vi "WPI_IMU_ADIS16448_Loop.vi"(8 "error in":errorcluster, 11 "ADI IMU Interrupt DevRef":T1={"ADI IMU DevRef"={"DevStatus"={"status"=FALSE, "code"=0, "source"=""}, "Handle"=0, "SPI Bus"=enum."SPI On-Board, CS0", "Device Found"=FALSE, "Device Ready"=FALSE, "Yaw Axis"=enum."Z", "AHRS Algorithm"=enum."Complementary", "Serial"=0, "Lot ID 2"=0, "Lot ID 1"=0, "Product ID"=0}, "InterruptRef"={"DevStatus"={"status"=FALSE, "code"=0, "source"=""}, "InterruptIndex"=enum."0"}}) -> (0 "error out":errorcluster, 1 "Device Found":bool)   [LabVIEW 2015, in "Apple Pi Gyro Library.lvlib" / "FRC_ADIS16448_IMU.lvlib"]
doc: "Periodically reads the ADI MXP IMU valuse and makes data available for use elsewhere in your robot project. Place this block within PeriodicTasks.vi outside any loops."
uses:
  FRC_ADIS16448_IMU.lvlib
  WPI_IMU_ADIS16448_InterruptDevRef.ctl
  WPI_IMU_ADIS16448_IMUDevRef.ctl
  <vilib>/Rock Robotics/SystemInterfaces/spilib/spi_bus.ctl
  <vilib>/Rock Robotics/WPI/Interrupt/WPI_InterruptRef.ctl
  <vilib>/Rock Robotics/SystemInterfaces/Interrupt/FPGA_InterruptIndex.ctl
  <vilib>/Rock Robotics/WPI/SPI/WPI_SPIDevRef.ctl
  WPI_IMU_ADIS16448_Registers.ctl
  <vilib>/Platform/TimedLoop/XDataNode/timing_clust.ctl
  <vilib>/Platform/TimedLoop/XDataNode/nitl_modes.ctl
  <vilib>/Platform/TimedLoop/XDataNode/wakeup.ctl
  <vilib>/Rock Robotics/SystemInterfaces/Utilities/FPGA_UtilitiesRead LocalTime.vi
  <vilib>/Rock Robotics/SystemInterfaces/Interrupt/FPGA_WaitOnInterrupt.vi
  <vilib>/Rock Robotics/WPI/Utilities/WPI_UtilitiesTimebaseConstants.vi
  <vilib>/Rock Robotics/SystemInterfaces/Interrupt/FPGA_InterruptReadTimestamp.vi
  <vilib>/platform/TimedLoop/XDataNode/XDataNode.xnode
  <vilib>/Platform/TimedLoop/XDataNode/XDNodeRunTimeDep.lvlib
  <vilib>/ptbypt/NI_PtbyPt.lvlib
panel:
  out "SPS":dbl
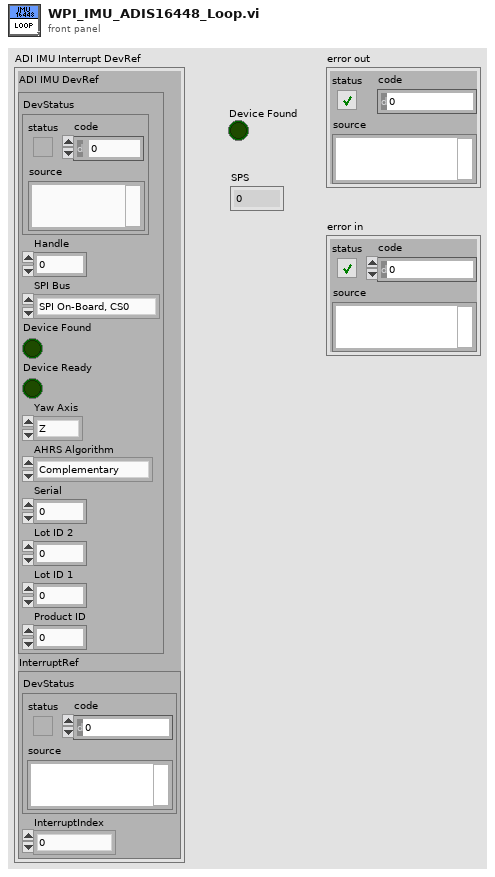
[diagram p1: front panel]
types:
  T1 = typedef "Apple Pi Gyro Library.lvlib/FRC_ADIS16448_IMU.lvlib/WPI_IMU_ADIS16448_InterruptDevRef.ctl" = cluster{"ADI IMU DevRef":T2, "InterruptRef":T4}
  T2 = typedef "Apple Pi Gyro Library.lvlib/FRC_ADIS16448_IMU.lvlib/WPI_IMU_ADIS16448_IMUDevRef.ctl" = cluster{"DevStatus":errorcluster, "Handle":i32, "SPI Bus":T3, "Device Found":bool, "Device Ready":bool, "Yaw Axis":enum16{"X", "Y", "Z"}, "AHRS Algorithm":enum16{"Complementary", "Madgwick"}, "Serial":u16, "Lot ID 2":u16, "Lot ID 1":u16, "Product ID":u16}
  T3 = typedef "spi_bus.ctl" = enum16{"SPI On-Board, CS0", "SPI On-Board, CS1", "SPI On-Board, CS2", "SPI On-Board, CS3", "SPI MXP", "Invalid"}
  T4 = typedef "WPI_InterruptRef.ctl" = cluster{"DevStatus":errorcluster, "InterruptIndex":T5}
  T5 = typedef "FPGA_InterruptIndex.ctl" = enum8{"0", "1", "2", "3", "4", "5", "6", "7", "Invalid"}
  T6 = typedef "WPI_SPIDevRef.ctl" = cluster{"DevStatus":errorcluster, "Handle":i32, "SPI Bus":T3}
  T7 = cluster{"read mode":enum16{"polling", "blocking"}, "write mode":enum16{"polling", "blocking"}}
  T8 = cluster{"X Angle":dbl, "Y Angle":dbl, "Z Angle":dbl}
  T9 = typedef "XDNodeRunTimeDep.lvlib/timing_clust.ctl" = cluster{"Expected End [f-1]":u64, "Actual End [f-1]":u64, "Finished Late? [f-1]":bool, "Expected End [i-1]":u64, "Actual End [i-1]":u64, "Finished Late? [i-1]":bool, "Expected Start [i]":u64, "Actual Start [i]":u64, "Expected Start [f]":u64, "Actual Start [f]":u64, "Source Name":string, "Structure Name":string, "Period":i64, "Deadline":i64, "Offset":i64, "Start":i64, "Priority":i32, "Timeout":i32, "Mode":T10, "Wakeup Reason":T11, "Error":errorcluster, "Source Type":string, "Secondary Source Type":string, "Global End Time":u64, "Global Start Time":u64, "Frame Duration":u64, "Iteration Duration":u64, "Assigned CPU":i32, "I/O Scan Engine Mode":u32}
  T10 = typedef "XDNodeRunTimeDep.lvlib/nitl_modes.ctl" = enum32{"No Change", "Process missed periods, maintain original phase", "Discard missed periods, maintain original phase", "Process missed periods, ignore original phase", "Discard missed periods, ignore original phase"}
  T11 = typedef "XDNodeRunTimeDep.lvlib/wakeup.ctl" = enum32{"Normal", "Aborted", "Asynchronous wakeup", "Timing source error", "Timed loop error", "Timeout"}
  T12 = cluster{"X Gyro":dbl, "Y Gyro":dbl, "Z Gyro":dbl, "X Accel":dbl, "Y Accel":dbl, "Z Accel":dbl, "X Mag":dbl, "Y Mag":dbl, "Z Mag":dbl, "Pressure":dbl, "Temp":dbl}
  T13 = typedef "Apple Pi Gyro Library.lvlib/FRC_ADIS16448_IMU.lvlib/WPI_IMU_ADIS16448_Registers.ctl" = u8
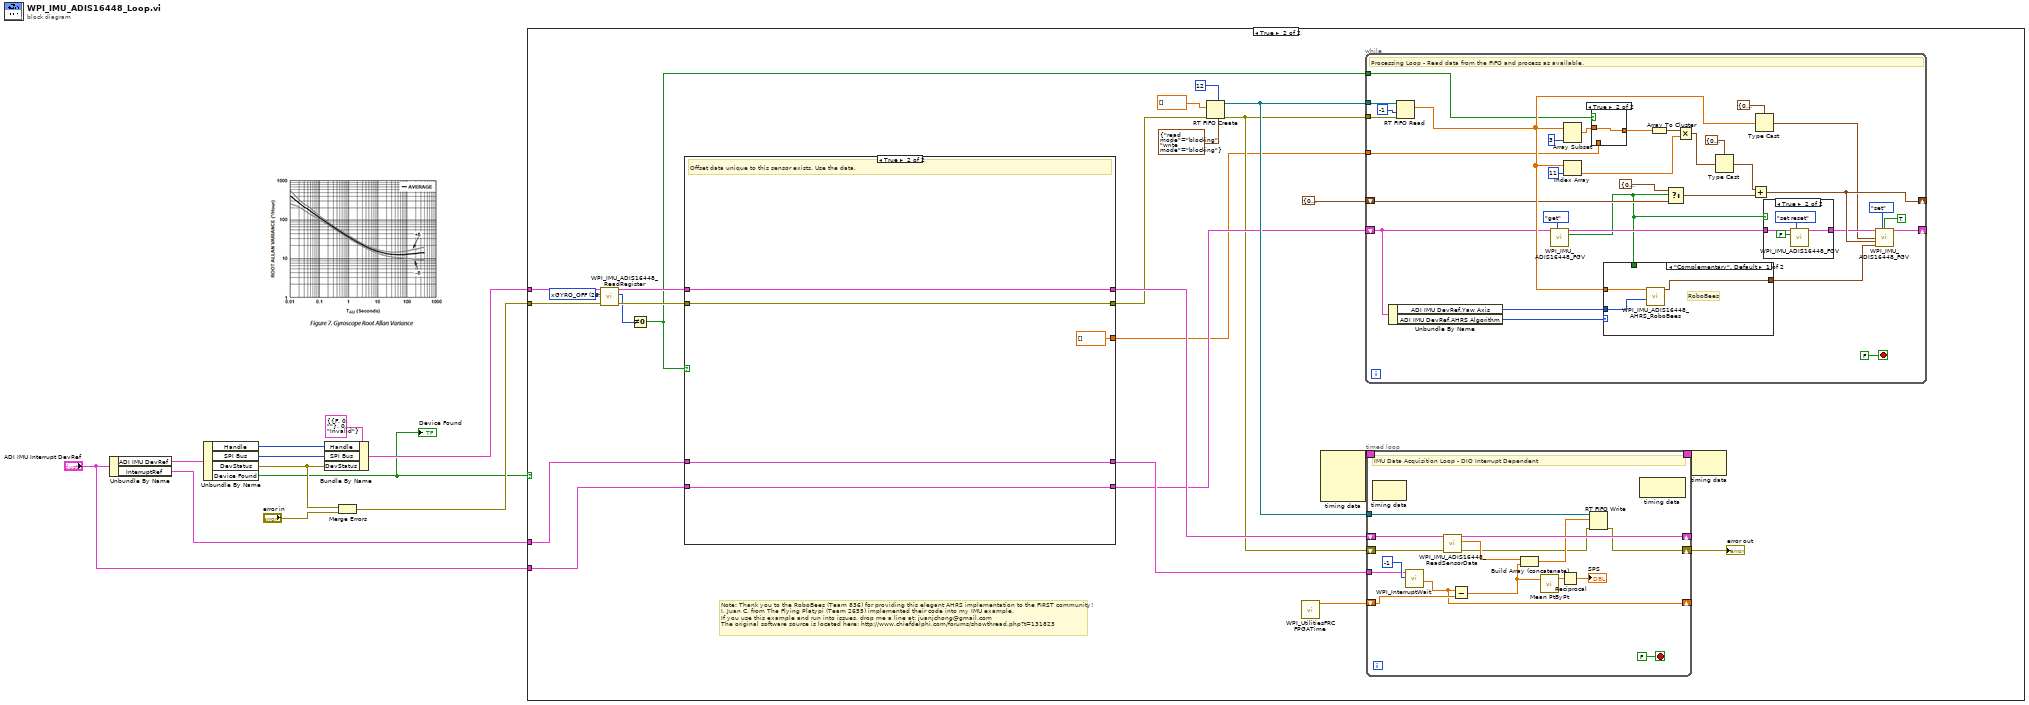
[diagram p0: block diagram]
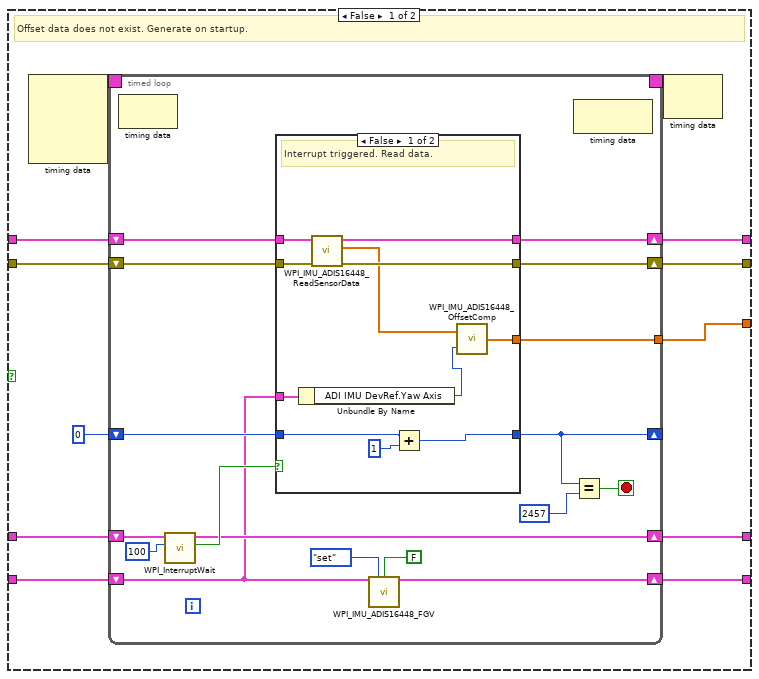
[diagram p3: hidden frame]
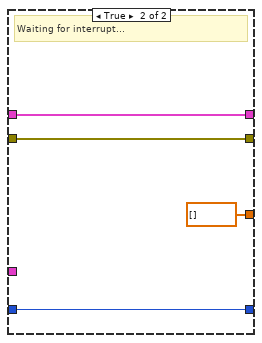
[diagram p4: hidden frame]
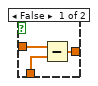
[diagram p5: hidden frame]
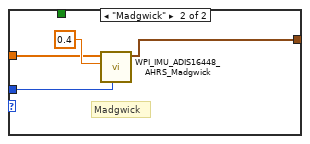
[diagram p6: hidden frame]
diagram:
  n1 = Unbundle By Name("ADI IMU Interrupt DevRef") -> ("ADI IMU DevRef"=w7:T2, "InterruptRef"=w3:T4)
  n2 = Unbundle By Name(w7) -> ("Handle"=w10:i32, "SPI Bus"=w9:T3, "DevStatus"=w8:errorcluster, "Device Found"=w1:bool)
  "Device Found" <- w1
  n3 = Bundle By Name(cluster=T6 {"DevStatus"={"status"=FALSE, "code"=0, "source"=""}, "Handle"=0, "SPI Bus"=enum."Invalid"} ("SPIDevRef out"), "Handle"=w10, "SPI Bus"=w9, "DevStatus"=w8) -> (w5:T6)
  n4 = Merge Errors(w8, "error in") -> (w4:errorcluster)
  n5 = case shown="True" w1 {
    tunnel: w5 -> [_ w21]
    tunnel: w4 -> [_ w20]
    tunnel: w3 -> [_ w31]
    tunnel: "ADI IMU Interrupt DevRef" -> [_ w30]
    frame False {
    }
    frame True {
      w17 = T13 26 items=["zGYRO_OFF"=30, "yGYRO_OFF"=28, "xGYRO_OFF"=26, "GLOB_CMD"=62, "SEQ_CNT"=58, "SMPL_PRD"=54, "SENS_AVG"=56, "MSC_CTRL"=52, "zACCEL_OFF"=36, "yACCEL_OFF"=34, "xACCEL_OFF"=32, "ERROR_FLAGS"=60, "TEMP"=24, "BARO"=22, "Z_MAG"=20, "Y_MAG"=18, "X_MAG"=16, "Z_ACCEL"=14, "Y_ACCEL"=12, "X_ACCEL"=10, "Z_GYRO"=8, "Y_GYRO"=6, "X_GYRO"=4, "PROD_ID"=86, "LOT_ID2"=84, "LOT_ID1"=82, "SERIAL_NUM"=88] ("ADIS16448 Register")
      # "Note: Thank you to the RoboBees (Team 836) for providing this elegant AHRS implementation to the FIRST community!\nI, Juan C. from The Flying Platypi (Team 2655) implemented their code into my IMU example.\nIf you use this example and run into issues, drop me a line at: juanjchong@gmail.com\nThe original software source is located here: http://www.chiefdelphi.com/forums/showthread.php?t=131823"
      n6 = call "WPI_IMU_ADIS16448_ReadRegister.vi"("error in (no error)"=w20, "ADIS16448 Register"=w17, "SPIDevRef in"=w21) -> ("error out"=w18:errorcluster, "Register Value"=w16:u16, "SPIDevRef out"=w19:T6)  [unwired: 6 in]
      n7 = Not Equal To 0?(x=w16) -> (x != 0?=w15:bool)
      n8 = case shown="True" w15 {
        tunnel: w19 -> [w64 w108]
        tunnel: w18 -> [w63 w107]
        tunnel: [w62 w108] -> w32
        tunnel: w31 -> [w61 w106]
        tunnel: w30 -> [w60 w105]
        tunnel: [w59 w106] -> w29
        tunnel: [w58 w105] -> w28
        tunnel: [w57 w107] -> w27
        tunnel: [w56 dbl[] [] ("Offset Compensated Data")] -> w22
        frame False {
          # "Offset data does not exist. Generate on startup."
          n9 = node-c288() -> (w67:T9)  [unwired: 4 in]
          n10 = timed-loop {
            shift-right: [w83] -> w62
            shift-left: w64 -> [w79]
            shift-right: [w84] -> w57
            shift-left: w63 -> [w78]
            shift-right: [w75] -> _
            shift-left: 0 -> [w82]
            timing: w67 -> [_]
            timing-out: [_] -> w66
            shift-right: [w72] -> w59
            shift-left: w61 -> [w73]
            shift-right: [w71] -> w58
            shift-left: w60 -> [w68]
            tunnel: [w69] -> w56
            stop <- w74 stop-if-true
            n11 = node-c288() -> ()  [unwired: 1 in, 1 out]
            n12 = call <vilib>:"WPI_InterruptWait.vi"("Timeout (ms)"=100, "InterruptRef"=w73) -> ("Timed Out"=w80:bool, "InterruptRef"=w72:T4)  [unwired: 5 in, 3 out]
            n13 = case shown="False" w80 {
              tunnel: [w97 w99] -> w84
              tunnel: [w96 w100] -> w83
              tunnel: w78 -> [w95 w99]
              tunnel: w79 -> [w94 w100]
              tunnel: w82 -> [w91 w101]
              tunnel: [w93 w101] -> w75
              tunnel: [w89 dbl[] [] ("Offset Compensated Data")] -> w69
              tunnel: w68 -> [w88 _]
              frame False {
                # "Interrupt triggered. Read data."
                n14 = Unbundle By Name(w88) -> ("ADI IMU DevRef.Yaw Axis"=w87:enum16{"X", "Y", "Z"})
                n15 = call "WPI_IMU_ADIS16448_ReadSensorData.vi"("error in (no error)"=w95, "SPIDevRef in"=w94) -> ("error out"=w97:errorcluster, "Data Array"=w90:dbl[], "SPIDevRef out"=w96:T6)  [unwired: 7 in]
                n16 = Add(x=w91, y=1) -> (x+y=w93:i32)
                n17 = call "WPI_IMU_ADIS16448_OffsetComp.vi"("Yaw Axis"=w87, "Raw Data"=w90) -> ("Offset Compensated Data"=w89:dbl[])
              }
              frame True {
                # "Waiting for interrupt..."
              }
            }
            n18 = call "WPI_IMU_ADIS16448_FGV.vi"("ADI IMU Interrupt DevRef"=w68, "Operation"=enum16{"set", "get", "set reset"}."set", "Sensor Ready?"=FALSE) -> ("ADI IMU Interrupt DevRef Out"=w71:T1)  [unwired: 6 in, 6 out]
            n19 = node-c288() -> ()  [unwired: 1 in, 1 out]
            n20 = Equal?(x=w75, y=2457) -> (x = y?=w74:bool)
          }
          n21 = node-c288(w66) -> ()  [unwired: 1 out]
        }
        frame True {
          # "Offset data unique to this sensor exists. Use the data."
        }
      }
      n22 = RT FIFO Create(1:dbl[] [] ("appended array"), 3:w27, 6:u32 12 ("elements in array (1)"), 7:T7 {"read mode"=enum."blocking", "write mode"=enum."blocking"} ("r/w modes (polling,polling)")) -> (8:w35:refnum<k33>, 11:w26:errorcluster)  [unwired: 4 in, 1 out]
      n23 = call <vilib>:"WPI_UtilitiesFRC FPGATime.vi"() -> ("FPGA Time"=w14:dbl)  [unwired: 10 in, 1 out]
      n24 = node-c288() -> (w13:T9)  [unwired: 4 in]
      n25 = while {
        tunnel: w35 -> [w140]
        shift-right: [w136] -> _
        shift-left: T8 {"X Angle"=0.0, "Y Angle"=0.0, "Z Angle"=0.0} ("IMU Angles") -> [w137]
        shift-right: [w133] -> _
        shift-left: w28 -> [w132]
        tunnel: w22 -> [w131]
        tunnel: w26 -> [w139]
        tunnel: w15 -> [w109]
        stop <- FALSE stop-if-true
        # "Processing Loop - Read data from the FIFO and process as available."
        n26 = Unbundle By Name(w132) -> ("ADI IMU DevRef.Yaw Axis"=w135:enum16{"X", "Y", "Z"}, "ADI IMU DevRef.AHRS Algorithm"=w134:enum16{"Complementary", "Madgwick"})
        n27 = RT FIFO Read(0:w140, 2:-1 ("timeout in ms (0)"), 3:w139) -> (9:w138:dbl[])  [unwired: 1 in, 4 out]
        n28 = call "WPI_IMU_ADIS16448_FGV.vi"("ADI IMU Interrupt DevRef"=w132, "Operation"=enum16{"set", "get", "set reset"}."get") -> ("ADI IMU Interrupt DevRef Out"=w116:T1, "Reset Out"=w111:bool)  [unwired: 7 in, 5 out]
        n29 = Array Subset(array=w138, length=3) -> (w128:dbl[])  [unwired: 1 in]
        n30 = Index Array(array=w138, index=11) -> (element=w115:dbl)
        n31 = case shown="True" w109 {
          tunnel: w131 -> [w144 _]
          tunnel: w128 -> [w143 w145]
          tunnel: [w142 w145] -> w127
          frame False {
            n32 = Subtract(x=w143, y=w144) -> (x-y=w142:dbl[])
          }
          frame True {
          }
        }
        n33 = case shown="\"Complementary\", Default" w134 {
          tunnel: w138 -> [w148 w151]
          tunnel: w135 -> [w147 w150]
          tunnel: w111 -> [_ _]
          tunnel: [w146 w149] -> w110
          frame "Complementary", Default {
            # "RoboBees"
            n34 = call "WPI_IMU_ADIS16448_AHRS_RoboBees.vi"("Yaw Axis"=w147, "IMU Rates"=w148) -> ("Output"=w146:cluster{"Pitch":dbl, "Roll":dbl, "Yaw":dbl})  [unwired: 5 in, 3 out]
          }
          frame "Madgwick" {
            # "Madgwick"
            n35 = call "WPI_IMU_ADIS16448_AHRS_Madgwick.vi"("Yaw Axis"=w150, "Beta"=0.4, "Data"=w151) -> ("Output"=w149:cluster{"Pitch":dbl, "Roll":dbl, "Yaw":dbl})  [unwired: 8 in]
          }
        }
        n36 = Array To Cluster(array=w127) -> (cluster=w126:cluster{"[0]":dbl, "[1]":dbl, "[2]":dbl})
        n37 = Select(t=T8 {"X Angle"=0.0, "Y Angle"=0.0, "Z Angle"=0.0} ("IMU Angles"), s=w111, f=w137) -> (s? t:f=w124:T8)
        n38 = Multiply(x=w126, y=w115) -> (x*y=w119:cluster{"[0]":dbl, "[1]":dbl, "[2]":dbl})
        n39 = Type Cast(type=T8 {"X Angle"=0.0, "Y Angle"=0.0, "Z Angle"=0.0} ("IMU Angles"), x=w119) -> (*(type *) &x=w120:T8)
        n40 = Add(x=w120, y=w124) -> (x+y=w136:T8)
        n41 = Type Cast(type=T12 {"X Gyro"=0.0, "Y Gyro"=0.0, "Z Gyro"=0.0, "X Accel"=0.0, "Y Accel"=0.0, "Z Accel"=0.0, "X Mag"=0.0, "Y Mag"=0.0, "Z Mag"=0.0, "Pressure"=0.0, "Temp"=0.0} ("IMU Data"), x=w138) -> (*(type *) &x=w113:T12)
        n42 = case shown="True" w111 {
          tunnel: [w153 w156] -> w117
          tunnel: w116 -> [w153 w155]
          frame False {
          }
          frame True {
            n43 = call "WPI_IMU_ADIS16448_FGV.vi"("ADI IMU Interrupt DevRef"=w155, "Operation"=enum16{"set", "get", "set reset"}."set reset", "Reset"=FALSE) -> ("ADI IMU Interrupt DevRef Out"=w156:T1)  [unwired: 6 in, 6 out]
          }
        }
        n44 = call "WPI_IMU_ADIS16448_FGV.vi"("ADI IMU Interrupt DevRef"=w117, "Operation"=enum16{"set", "get", "set reset"}."set", "Sensor Ready?"=TRUE, "IMU Data"=w113, "IMU Angles"=w136, "IMU AHRS"=w110) -> ("ADI IMU Interrupt DevRef Out"=w133:T1)  [unwired: 3 in, 6 out]
      }
      n45 = timed-loop {
        tunnel: w35 -> [w50]
        shift-right: [w46] -> _
        shift-left: w32 -> [w48]
        shift-right: [w45] -> w25
        shift-left: w26 -> [w47]
        tunnel: w29 -> [w44]
        shift-right: [w42] -> _
        shift-left: w14 -> [w43]
        timing: w13 -> [_]
        timing-out: [_] -> w12
        stop <- FALSE stop-if-true
        # "IMU Data Acquisition Loop - DIO Interrupt Dependent"
        n46 = node-c288() -> ()  [unwired: 1 in, 1 out]
        n47 = call <vilib>:"WPI_InterruptWait.vi"("Timeout (ms)"=-1, "InterruptRef"=w44) -> ("TimeStamp"=w42:dbl)  [unwired: 5 in, 4 out]
        n48 = call "WPI_IMU_ADIS16448_ReadSensorData.vi"("error in (no error)"=w47, "SPIDevRef in"=w48) -> ("error out"=w39:errorcluster, "Data Array"=w41:dbl[], "SPIDevRef out"=w46:T6)  [unwired: 7 in]
        n49 = Subtract(x=w42, y=w43) -> (x-y=w38:dbl)
        n50 = Build Array (concatenate)(w41, w38) -> (w40:dbl[])
        n51 = call <vilib>:"Mean PtByPt.vi"("x"=w38) -> ("mean"=w37:dbl)  [unwired: 3 in, 1 out]
        n52 = Reciprocal(x=w37) -> (1/x=→"SPS":dbl)
        n53 = RT FIFO Write(0:w50, 1:w40, 3:w39) -> (11:w45:errorcluster)  [unwired: 2 in, 3 out]
        n54 = node-c288() -> ()  [unwired: 1 in, 1 out]
      }
      "error out" <- w25
      n55 = node-c288(w12) -> ()  [unwired: 1 out]
    }
  }
